vi "Lang.Pro.vi"(6 "Value_In_4_cn?":bool, 7 "lang":enum16{"zh", "en", "it"}(ring), 8 "error in (no error)":errorcluster caption="错误输入（无错误）", 9 "value in":string caption="Value In", 10 "key":string caption="Key", 11 "基路径":path) -> (0 "error out":errorcluster caption="错误输出", 1 "value out":string caption="Value Out", 3 "Find?":bool)   [LabVIEW 2012, in "Lib_UEL.ATE.lvlib" / "Lib_App.lvlib"]
uses:
  Lib_App.lvlib
  <vilib>/Utility/config.llb/Read Key (String).vi
  <vilib>/Utility/config.llb/Write Key (String).vi
  <vilib>/Utility/config.llb/NI_LVConfig.lvlib
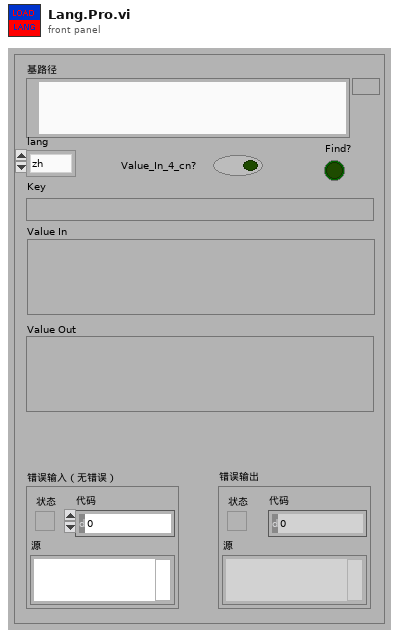
[diagram p1: front panel]
types:
  T1 = typedef "NI_LVConfig.lvlib/Config Data RefNum.ctl" = refnum<k1>
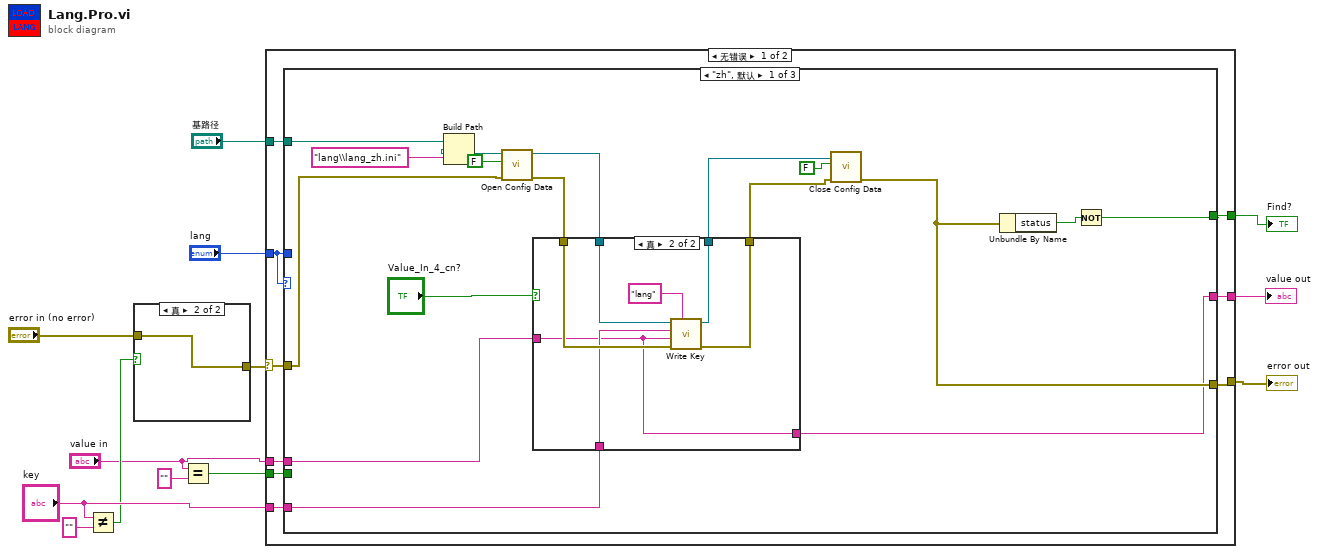
[diagram p0: block diagram]
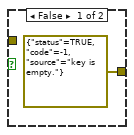
[diagram p2: hidden frame]
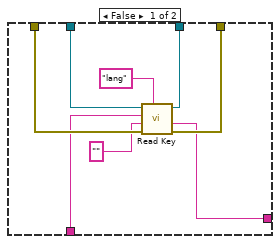
[diagram p3: hidden frame]
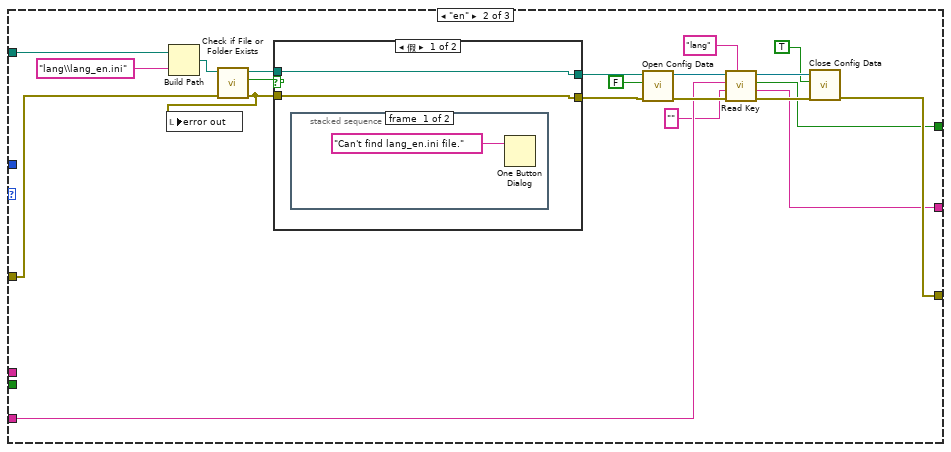
[diagram p4: hidden frame]
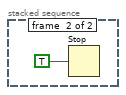
[diagram p5: hidden frame]
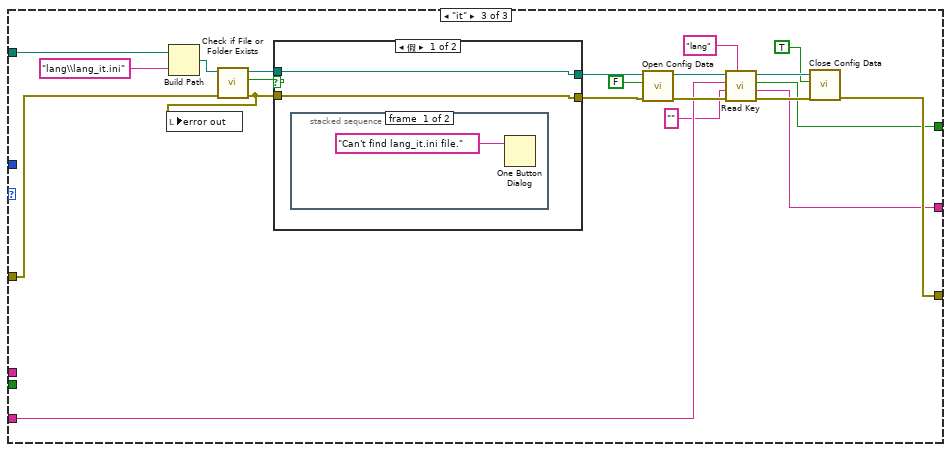
[diagram p7: hidden frame]
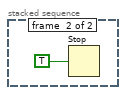
[diagram p8: hidden frame]
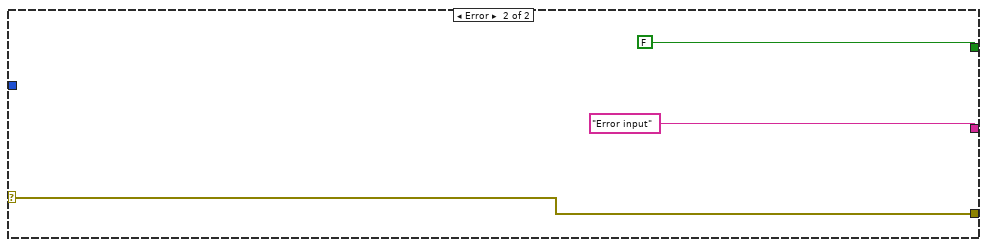
[diagram p10: hidden frame]
diagram:
  n1 = Not Equal?(x="key", y="") -> (x != y?=w6:bool)
  n2 = case shown="真" w6 {
    tunnel: [errorcluster {"status"=TRUE, "code"=-1, "source"="key is empty."} ("error IO") w15] -> w5
    tunnel: "error in (no error)" -> [_ w15]
    frame False {
    }
    frame True {
    }
  }
  n3 = Equal?(x="value in", y="") -> (x = y?=w1:bool)
  n4 = case shown="无错误" w5 {
    selector: w5 -> [w23 w113]
    tunnel: "基路径" -> [w24 _]
    tunnel: "lang" -> [w18 _]
    tunnel: [w19 w113] -> w11
    tunnel: "key" -> [w21 _]
    tunnel: [w22 "Error input" ("value")] -> w10
    tunnel: [w20 FALSE ("found?")] -> w9
    tunnel: "value in" -> [w17 _]
    tunnel: w1 -> [w16 _]
    frame No Error {
      n5 = case shown="\"zh\", 默认" w18 {
        tunnel: w18 -> [_ _ _]
        tunnel: w24 -> [w40 w74 w101]
        tunnel: w23 -> [w36 w64 w91]
        tunnel: [w26 w58 w85] -> w22
        tunnel: w21 -> [w28 w60 w87]
        tunnel: [w33 w57 w84] -> w20
        tunnel: [w35 w61 w88] -> w19
        tunnel: w17 -> [w27 _ _]
        tunnel: w16 -> [_ _ _]
        frame "zh", Default {
          n6 = Build Path(base path=w40, name or relative path="lang\\lang_zh.ini" ("名称或相对路径")) -> (appended path=w37:path)
          n7 = call <vilib>:"Open Config Data.vi"("error in (no error)"=w36, "create file if necessary (T)"=FALSE ("create file if necessary? (T)"), "configuration file path"=w37) -> ("error out"=w31:errorcluster, "refnum"=w32:T1)  [unwired: 6 in, 1 out]
          n8 = case shown="真" "Value_In_4_cn?" {
            tunnel: w32 -> [w48 w55]
            tunnel: w31 -> [w47 w54]
            tunnel: [w46 w53] -> w30
            tunnel: [w45 w52] -> w29
            tunnel: w28 -> [w44 w51]
            tunnel: w27 -> [_ w50]
            tunnel: [w43 w50] -> w26
            frame False {
              n9 = call-poly <vilib>:"Read Key.vi"("section"="lang", "error in (no error)"=w47, "default value"="" ("y"), "key"=w44, "refnum"=w48) -> ("error out"=w45:errorcluster, "value"=w43:string, "refnum out"=w46:T1)  [unwired: 3 in, 1 out]
            }
            frame True {
              n10 = call-poly <vilib>:"Write Key.vi"("section"="lang", "error in (no error)"=w54, "value"=w50, "key"=w51, "refnum"=w55) -> ("error out"=w52:errorcluster, "refnum out"=w53:T1)  [unwired: 4 in, 1 out]
            }
          }
          n11 = call <vilib>:"Close Config Data.vi"("error in (no error)"=w29, "write file if changed (T)"=FALSE ("write configuration file? (T)"), "refnum"=w30) -> ("error out"=w35:errorcluster)  [unwired: 7 in, 1 out]
          n12 = Unbundle By Name(w35) -> ("status"=w34:bool)
          n13 = Not(x=w34) -> (.not. x?=w33:bool)
        }
        frame "en" {
          n14 = Build Path(base path=w74, name or relative path="lang\\lang_en.ini" ("名称或相对路径")) -> (appended path=w76:path)
          n15 = call <vilib>:"Check if File or Folder Exists.vi"("error in (no error)"=w64, "path"=w76) -> ("error out"=w62:errorcluster, "file or folder exists?"=w75:bool, "dup path"=w73:path)  [unwired: 7 in]
          n16 = local write "error out"(w62) -> ()
          n17 = case shown="假" w75 {
            tunnel: [w79 w83] -> w72
            tunnel: w73 -> [w79 w83]
            tunnel: [w78 w82] -> w63
            tunnel: w62 -> [w78 w82]
            frame False {
              n18 = stacked-sequence {
                frame #0 {
                  n19 = One Button Dialog(message="Can't find lang_en.ini file." ("消息")) -> ()  [unwired: 1 in, 1 out]
                }
                frame #1 {
                  n20 = Stop(stop? (T)=TRUE ("停止？(T)")) -> ()
                }
              }
            }
            frame True {
            }
          }
          n21 = call <vilib>:"Open Config Data.vi"("error in (no error)"=w63, "create file if necessary (T)"=FALSE ("create file if necessary? (T)"), "configuration file path"=w72) -> ("error out"=w69:errorcluster, "refnum"=w70:T1)  [unwired: 6 in, 1 out]
          n22 = call-poly <vilib>:"Read Key.vi"("section"="lang", "error in (no error)"=w69, "default value"="" ("section"), "key"=w60, "refnum"=w70) -> ("error out"=w66:errorcluster, "value"=w58:string, "found?"=w57:bool, "refnum out"=w67:T1)  [unwired: 3 in]
          n23 = call <vilib>:"Close Config Data.vi"("error in (no error)"=w66, "write file if changed (T)"=TRUE ("write configuration file? (T)"), "refnum"=w67) -> ("error out"=w61:errorcluster)  [unwired: 7 in, 1 out]
        }
        frame "it" {
          n24 = Build Path(base path=w101, name or relative path="lang\\lang_it.ini" ("名称或相对路径")) -> (appended path=w103:path)
          n25 = call <vilib>:"Check if File or Folder Exists.vi"("error in (no error)"=w91, "path"=w103) -> ("error out"=w89:errorcluster, "file or folder exists?"=w102:bool, "dup path"=w100:path)  [unwired: 7 in]
          n26 = local write "error out"(w89) -> ()
          n27 = case shown="假" w102 {
            tunnel: [w106 w110] -> w99
            tunnel: w100 -> [w106 w110]
            tunnel: [w105 w109] -> w90
            tunnel: w89 -> [w105 w109]
            frame False {
              n28 = stacked-sequence {
                frame #0 {
                  n29 = One Button Dialog(message="Can't find lang_it.ini file." ("消息")) -> ()  [unwired: 1 in, 1 out]
                }
                frame #1 {
                  n30 = Stop(stop? (T)=TRUE ("停止？(T)")) -> ()
                }
              }
            }
            frame True {
            }
          }
          n31 = call <vilib>:"Open Config Data.vi"("error in (no error)"=w90, "create file if necessary (T)"=FALSE ("create file if necessary? (T)"), "configuration file path"=w99) -> ("error out"=w96:errorcluster, "refnum"=w97:T1)  [unwired: 6 in, 1 out]
          n32 = call-poly <vilib>:"Read Key.vi"("section"="lang", "error in (no error)"=w96, "default value"="" ("section"), "key"=w87, "refnum"=w97) -> ("error out"=w93:errorcluster, "value"=w85:string, "found?"=w84:bool, "refnum out"=w94:T1)  [unwired: 3 in]
          n33 = call <vilib>:"Close Config Data.vi"("error in (no error)"=w93, "write file if changed (T)"=TRUE ("write configuration file? (T)"), "refnum"=w94) -> ("error out"=w88:errorcluster)  [unwired: 7 in, 1 out]
        }
      }
    }
    frame Error {
    }
  }
  "error out" <- w11
  "value out" <- w10
  "Find?" <- w9
